vi "FilePath.vi"() -> ()   [LabVIEW 2017]
panel:
  in  "Path":path
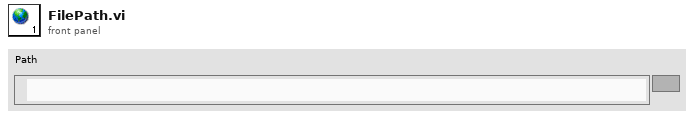
[diagram p1: front panel]
diagram:
